vi "Monitor_Lithography_DAQ.vi"(8 "error in":errorcluster, 9 "Bmp Path":string, 10 "DAQ Channel":tag="Dev4/ai0:3", 11 "Application":refnum<k7>) -> (0 "error out":errorcluster)   [LabVIEW 2016]
panel:
  out "Tip Voltage":dbl
  out "Stop?":bool
  out "Position":cluster{dbl[], dbl[]}[](graph)=[{[8.144911482214924], [8.14400435631275]}, {[8.144911482214924, 8.144910315132138], [8.14400435631275, 8.144007987236977]}, {[8.144910315132138, 8.144959851312642], [8.144007987236977, 8.14406716265678]}, {[8.144959851312642, 8.144927562022207], [8.14406716265678, 8.144052941536904]}, {[8.144927562022207, 8.144947143077852], [8.144052941536904, 8.144056140208242]}, {[8.144947143077852, 8.144929852962496], [8.144056140208242, 8.144053935718532]}, {[8.144929852962496, 8.144989676761625], [8.144053935718532, 8.144058776950834]}, {[8.144989676761625, 8.144944549560549], [8.144058776950834, 8.144003621482849]}, {[8.144944549560549, 8.144922936916354], [8.144003621482849, 8.14404416680336]}, {[8.144922936916354, 8.144971954393386], [8.14404416680336, 8.144050045442585]}, {[8.144971954393386, 8.144984921979903], [8.144050045442585, 8.144040665555]}, {[8.144984921979903, 8.144920170497892], [8.144040665555, 8.144028389573094]}, {[8.144920170497892, 8.144943468928338], [8.144028389573094, 8.144053935718535]}, {[8.144943468928338, 8.144931754875186], [8.144053935718535, 8.144048835134507]}, {[8.144931754875186, 8.144938930273055], [8.144048835134507, 8.143980884981152]}, {[8.144938930273055, 8.144918657612802], [8.143980884981152, 8.144049353837962]}, {[8.144918657612802, 8.144969274425508], [8.144049353837962, 8.144027827644347]}, {[8.144969274425508, 8.144959721636772], [8.144027827644347, 8.144028648924827]}, {[8.144959721636772, 8.144974461460114], [8.144028648924827, 8.144024067044258]}, {[8.144974461460114, 8.144973596954344], [8.144024067044258, 8.144094956517216]}, {[8.144973596954344, 8.144982803940772], [8.144094956517216, 8.144038936543465]}, {[8.144982803940772, 8.14491061770916], [8.144038936543465, 8.14405030479431]}, {[8.14491061770916, 8.144952243661878], [8.14405030479431, 8.14406543364525]}, {[8.144952243661878, 8.144953886222842], [8.14406543364525, 8.144027395391467]}, {[8.144953886222842, 8.144932749056816], [8.144027395391467, 8.143989875841138]}, {[8.144932749056816, 8.144925616884233], [8.143989875841138, 8.144035478520392]}, {[8.144925616884233, 8.14495777649879], [8.144035478520392, 8.1440280005455]}, {[8.14495777649879, 8.144938195443158], [8.1440280005455, 8.143993593215939]}, {[8.144938195443158, 8.144955442333218], [8.143993593215939, 8.144091714620592]}, {[8.144955442333218, 8.144975931119921], [8.144091714620592, 8.14405363314152]}, {[8.144975931119921, 8.14493832511902], [8.14405363314152, 8.14401408200264]}, {[8.14493832511902, 8.14495574491024], [8.14401408200264, 8.14406050596237]}, {[8.14495574491024, 8.144944203758241], [8.14406050596237, 8.144046025490757]}, {[8.144944203758241, 8.144971522140503], [8.144046025490757, 8.14400941367149]}, {[8.144971522140503, 8.144928469753266], [8.14400941367149, 8.14405065059662]}, {[8.144928469753266, 8.144966118979456], [8.14405065059662, 8.14405553505421]}, {[8.144966118979456, 8.144937806415557], [8.14405553505421, 8.14403526239395]}, {[8.144937806415557, 8.144933310985564], [8.14403526239395, 8.144018101954456]}, {[8.144933310985564, 8.14493387291431], [8.144018101954456, 8.14404498808384]}, {[8.14493387291431, 8.144930933594702], [8.14404498808384, 8.144022510933878]}, {[8.144930933594702, 8.144931841325759], [8.144022510933878, 8.14399752671718]}, {[8.144931841325759, 8.144960499691958], [8.14399752671718, 8.144025493478775]}, {[8.144960499691958, 8.144941307663915], [8.144025493478775, 8.144049267387388]}, {[8.144941307663915, 8.144946408247947], [8.144049267387388, 8.1440012008667]}, {[8.144946408247947, 8.144917231178281], [8.1440012008667, 8.144034916591643]}, {[8.144917231178281, 8.144966378331182], [8.144034916591643, 8.14403746688366]}, {[8.144966378331182, 8.14490841321945], [8.14403746688366, 8.144000077009201]}, {[8.14490841321945, 8.144950514650342], [8.144000077009201, 8.144042913269997]}, {[8.144950514650342, 8.144938973498343], [8.144042913269997, 8.144022251582141]}, {[8.144938973498343, 8.144915026688574], [8.144022251582141, 8.143997094464304]}, {[8.144915026688574, 8.144913427352902], [8.143997094464304, 8.144011920738215]}, {[8.144913427352902, 8.144943468928338], [8.144011920738215, 8.144038936543463]}, {[8.144943468928338, 8.144950774002075], [8.144038936543463, 8.144024542522432]}, {[8.144950774002075, 8.144900027513504], [8.144024542522432, 8.144039973950383]}, {[8.144900027513504, 8.144928988456723], [8.144039973950383, 8.144039195895196]}, {[8.144928988456723, 8.144915415716165], [8.144039195895196, 8.14405194735527]}, {[8.144915415716165, 8.14489765012264], [8.14405194735527, 8.14400024991035]}, {[8.14489765012264, 8.144920343399047], [8.14400024991035, 8.144039325571056]}, {[8.144920343399047, 8.144949693369865], [8.144039325571056, 8.144044253253933]}, {[8.144949693369865, 8.144898860430716], [8.144044253253933, 8.144037337207797]}, {[8.144898860430716, 8.14497679562569], [8.144037337207797, 8.144061413693427]}, {[8.14497679562569, 8.144909580302238], [8.144061413693427, 8.144041659736635]}, {[8.144909580302238, 8.14492168338299], [8.144041659736635, 8.144023159313202]}, {[8.14492168338299, 8.144926783967016], [8.144023159313202, 8.144075807714463]}, {[8.144926783967016, 8.144996376681332], [8.144075807714463, 8.144012007188797]}, {[8.144996376681332, 8.144929507160185], [8.144012007188797, 8.14405004544258]}, {[8.144929507160185, 8.145012413263322], [8.14405004544258, 8.14407943863869]}, {[8.145012413263322, 8.144946970176695], [8.14407943863869, 8.144047970628739]}, {[8.144946970176695, 8.144920645976068], [8.144047970628739, 8.144028994727133]}, {[8.144920645976068, 8.144951768183708], [8.144028994727133, 8.144036256575587]}, {[8.144951768183708, 8.144971478915213], [8.144036256575587, 8.144038979768757]}, {[8.144971478915213, 8.144902750706668], [8.144038979768757, 8.144039844274518]}, {[8.144902750706668, 8.144973251152038], [8.144039844274518, 8.144061975622176]}, {[8.144973251152038, 8.14498885548115], [8.144061975622176, 8.144065649771688]}, {[8.14498885548115, 8.144957387471196], [8.144065649771688, 8.144028259897231]}, {[8.144957387471196, 8.144947705006599], [8.144028259897231, 8.14407745027542]}, {[8.144947705006599, 8.144953929448127], [8.14407745027542, 8.144061024665831]}, {[8.144953929448127, 8.144903269410129], [8.144061024665831, 8.144016761970521]}, {[8.144903269410129, 8.144941653466221], [8.144016761970521, 8.144070318102834]}, {[8.144941653466221, 8.144920256948469], [8.144070318102834, 8.144042178440095]}, {[8.144920256948469, 8.144934391617772], [8.144042178440095, 8.144027308940883]}, {[8.144934391617772, 8.144905517125128], [8.144027308940883, 8.14404338874817]}, {[8.144905517125128, 8.144976190471647], [8.14404338874817, 8.144069410371785]}, {[8.144976190471647, 8.144912562847137], [8.144069410371785, 8.143993204188344]}, {[8.144912562847137, 8.144963698363302], [8.143993204188344, 8.14406513106823]}, {[8.144963698363302, 8.144939276075362], [8.14406513106823, 8.144064828491208]}, {[8.144939276075362, 8.144948007583617], [8.144064828491208, 8.144054886674885]}, {[8.144948007583617, 8.14492427690029], [8.144054886674885, 8.14402268383503]}, {[8.14492427690029, 8.144954102349281], [8.14402268383503, 8.144067076206207]}, {[8.144954102349281, 8.144972775673866], [8.144067076206207, 8.144025839281083]}, {[8.144972775673866, 8.144915761518481], [8.144025839281083, 8.144049526739119]}, {[8.144915761518481, 8.144925833010676], [8.144049526739119, 8.144036991405484]}, {[8.144925833010676, 8.14495820875168], [8.144036991405484, 8.144011315584184]}, {[8.14495820875168, 8.144922893691064], [8.144011315584184, 8.144008203363418]}, {[8.144922893691064, 8.144907678389552], [8.144008203363418, 8.144014211678504]}, {[8.144907678389552, 8.144932619380949], [8.144014211678504, 8.14401641616821]}, {[8.144932619380949, 8.144914464759827], [8.14401641616821, 8.14404101135731]}, {[8.144914464759827, 8.144949347567556], [8.14404101135731, 8.144062796902652]}, {[8.144949347567556, 8.14494070250988], [8.144062796902652, 8.144028778600694]}, {[8.14494070250988, 8.144930069088938], [8.144028778600694, 8.144016070365904]}, {[8.144930069088938, 8.144888788938522], [8.144016070365904, 8.144020392894745]}, {[8.144888788938522, 8.144961926126483], [8.144020392894745, 8.144041832637786]}, {[8.144961926126483, 8.1449480940342], [8.144041832637786, 8.143984386229514]}, {[8.1449480940342, 8.144913297677041], [8.143984386229514, 8.144037121081352]}, {[8.144913297677041, 8.144947402429576], [8.144037121081352, 8.144033274030681]}, {[8.144947402429576, 8.144933094859123], [8.144033274030681, 8.144044426155087]}, {[8.144933094859123, 8.144935774827], [8.144044426155087, 8.144036040449144]}, {[8.144935774827, 8.144959289383886], [8.144036040449144, 8.14409002883434]}, {[8.144959289383886, 8.144931971001627], [8.14409002883434, 8.144005955648424]}, {[8.144931971001627, 8.144940270256994], [8.144005955648424, 8.144060116934776]}, {[8.144940270256994, 8.14496897184849], [8.144060116934776, 8.144052941536904]}, {[8.14496897184849, 8.144953756546977], [8.144052941536904, 8.144020263218877]}, {[8.144953756546977, 8.144940961861613], [8.144020263218877, 8.144020695471761]}, {[8.144940961861613, 8.144948915314673], [8.144020695471761, 8.144057955670357]}, {[8.144948915314673, 8.144953281068803], [8.144057955670357, 8.14403707785606]}, {[8.144953281068803, 8.144914335083962], [8.14403707785606, 8.144033533382416]}, {[8.144914335083962, 8.144987299370765], [8.144033533382416, 8.144030766963962]}, {[8.144987299370765, 8.144963828039167], [8.144030766963962, 8.144050520920752]}, {[8.144963828039167, 8.144963482236864], [8.144050520920752, 8.144027006363867]}, {[8.144963482236864, 8.144932273578641], [8.144027006363867, 8.144054497647284]}, {[8.144932273578641, 8.144970700860023], [8.144054497647284, 8.144073214197158]}, {[8.144970700860023, 8.144905819702148], [8.144073214197158, 8.144001806020734]}, {[8.144905819702148, 8.144957646822926], [8.144001806020734, 8.144050002217293]}, {[8.144957646822926, 8.144944981813431], [8.144050002217293, 8.14404740869999]}, {[8.144944981813431, 8.144936898684502], [8.14404740869999, 8.14403798558712]}, {[8.144936898684502, 8.144909407401085], [8.14403798558712, 8.144014384579659]}, {[8.144909407401085, 8.144961623549463], [8.144014384579659, 8.14405328733921]}, {[8.144961623549463, 8.144910488033295], [8.14405328733921, 8.144024326395991]}, {[8.144910488033295, 8.144942517971996], [8.144024326395991, 8.144046155166626]}, {[8.144942517971996, 8.14495820875168], [8.144046155166626, 8.144048489332201]}, {[8.14495820875168, 8.14493344066143], [8.144048489332201, 8.14401598391533]}, {[8.14493344066143, 8.144943814730647], [8.14401598391533, 8.14403932557106]}, {[8.144943814730647, 8.144969836354253], [8.14403932557106, 8.144098284864423]}, {[8.144969836354253, 8.144990584492684], [8.144098284864423, 8.14402605540752]}, {[8.144990584492684, 8.144929852962496], [8.14402605540752, 8.144051212525367]}, {[8.144929852962496, 8.145005367541316], [8.144051212525367, 8.144065692996977]}, {[8.145005367541316, 8.144951811408996], [8.144065692996977, 8.14404386422634]}, {[8.144951811408996, 8.1449167989254], [8.14404386422634, 8.14404287004471]}, {[8.1449167989254, 8.144952157211304], [8.14404287004471, 8.14408687338829]}, {[8.144952157211304, 8.144971997618672], [8.14408687338829, 8.14401836130619]}]
  # "For Local Variables"
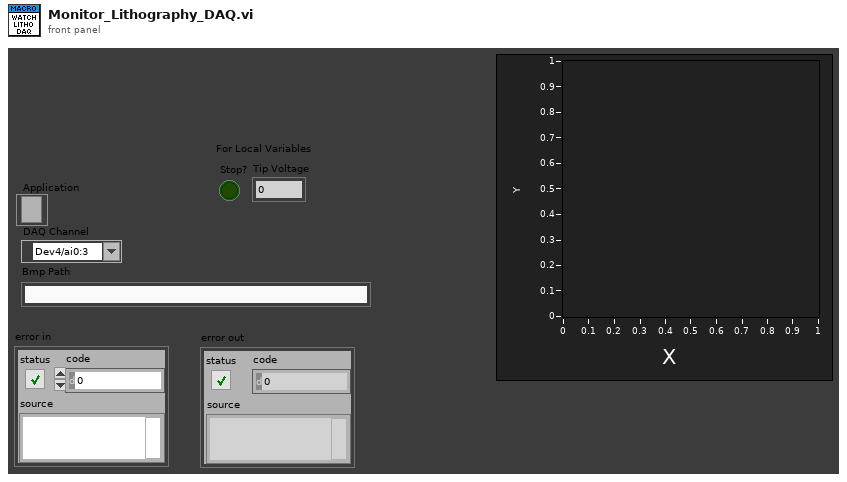
[diagram p1: front panel]
types:
  T1 = cluster{"Application":refnum<k7>, "Litho":refnum<k7>, "ZContr":refnum<k7>, "Scan":refnum<k7>}
  T2 = typedef "LVBoundsTypeDef.ctl" = cluster{"Width":u32, "Height":u32}
  T3 = typedef "LVPositionTypeDef.ctl" = cluster{"Left":i32, "Top":i32}
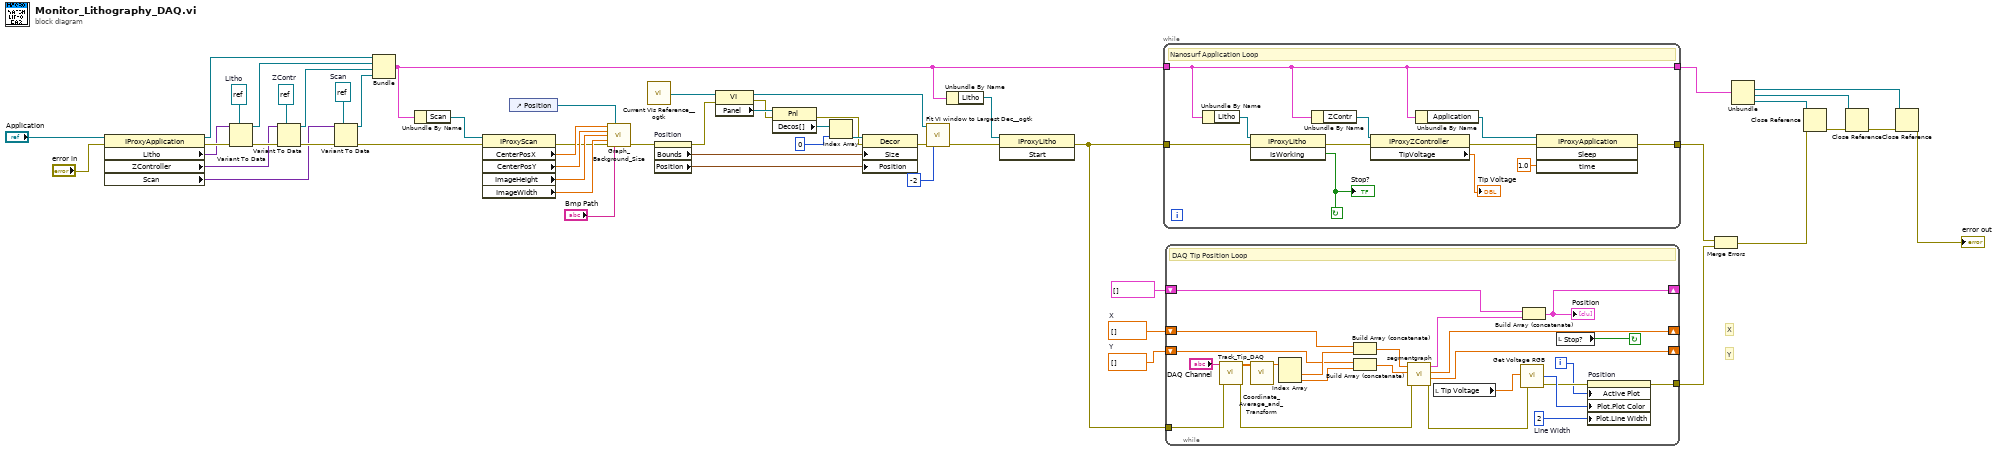
[diagram p0: block diagram]
diagram:
  w43 = dbl[] []  # Y
  w44 = dbl[] []  # X
  w46 = refnum<k7> refnum  # Scan
  w49 = refnum<k7> refnum  # ZContr
  w52 = refnum<k7> refnum  # Litho
  # "Y"
  # "X"
  n1 = property class="IProxyApplication"(reference="Application", error in="error in") -> (reference out=w36:refnum<k7>, error out=w54:errorcluster, "Litho"=w51:variant, "ZController"=w50:variant, "Scan"=w47:variant)
  n2 = Variant To Data(error in=w54, type=w52, Variant=w51) -> (data=w37:refnum<k7>, error out=w53:errorcluster)
  n3 = Variant To Data(error in=w53, type=w49, Variant=w50) -> (data=w35:refnum<k7>, error out=w48:errorcluster)
  n4 = Variant To Data(error in=w48, type=w46, Variant=w47) -> (data=w34:refnum<k7>, error out=w45:errorcluster)
  n5 = Bundle("Application"=w36, "Litho"=w37, "ZContr"=w35, "Scan"=w34) -> (w32:T1)  [unwired: 1 in]
  n6 = Unbundle By Name(w32) -> ("Scan"=w33:refnum<k7>)
  n7 = property class="IProxyScan"(reference=w33, error in=w45) -> (error out=w1:errorcluster, "CenterPosX"=w14:dbl, "CenterPosY"=w13:dbl, "ImageHeight"=w12:dbl, "ImageWidth"=w11:dbl)  [unwired: 1 out]
  n8 = control-ref of="Position"() -> (w15:refnum<vi>)
  n9 = call "Graph_Background_Size.vi"("CenterPosX"=w14, "XYGraph in"=w15, "CenterPosY"=w13, "Image Width"=w12, "Image Height"=w11, "error in (no error)"=w1, "Bmp Path"="Bmp Path") -> ("error out"=w17:errorcluster)  [unwired: 8 in]
  n10 = call <userlib>:"Current VIs Reference__ogtk.vi"() -> ("Current VI's reference"=w29:refnum<vi>)  [unwired: 5 in]
  n11 = property on="Position" class="XYGraph (strict)"(error in=w17) -> (error out=w20:errorcluster, "Bounds"=w24:T2, "Position"=w23:T3)  [unwired: 1 in, 1 out]
  n12 = property class="VI"(reference=w29, error in=w20) -> (reference out=w18:refnum<vi>, error out=w22:errorcluster, "Panel"=w28:refnum<vi>)
  n13 = property class="Pnl"(reference=w28, error in=w22) -> (error out=w21:errorcluster, "Decos[]"=w27:refnum<vi>[])  [unwired: 1 out]
  n14 = Index Array(array=w27, index=0) -> (element=w25:refnum<vi>)
  n15 = property class="Decor"(reference=w25, error in=w21, "Size"=w24, "Position"=w23) -> (error out=w19:errorcluster)  [unwired: 1 out]
  n16 = call <userlib>:"Fit VI window to Largest Dec__ogtk.vi"("error in (no error)"=w19, "border spacing (2 px)"=-2, "VI Ref (calling VI)"=w18) -> ("error out"=w16:errorcluster)  [unwired: 3 in, 1 out]
  n17 = Unbundle By Name(w32) -> ("Litho"=w31:refnum<k7>)
  n18 = invoke class="IProxyLitho" method="Start"(reference=w31, error in=w16) -> (error out=w41:errorcluster)  [unwired: 1 in, 2 out]
  n19 = while {
    tunnel: w41 -> [w66]
    tunnel: [w59] -> w39
    tunnel: w32 -> [w56]
    tunnel: [w56] -> w10
    stop <- w65 continue-if-true
    # "Nanosurf Application Loop"
    n20 = Unbundle By Name(w56) -> ("Litho"=w63:refnum<k7>)
    n21 = invoke class="IProxyLitho" method="IsWorking"(reference=w63, error in=w66) -> (error out=w64:errorcluster, "IsWorking"=w65:bool)  [unwired: 1 in, 1 out]
    "Stop?" <- w65
    n22 = Unbundle By Name(w56) -> ("ZContr"=w62:refnum<k7>)
    n23 = property class="IProxyZController"(reference=w62, error in=w64) -> (error out=w60:errorcluster, "TipVoltage"=→"Tip Voltage":dbl)  [unwired: 1 out]
    n24 = Unbundle By Name(w56) -> ("Application"=w58:refnum<k7>)
    n25 = invoke class="IProxyApplication" method="Sleep"(reference=w58, error in=w60, "time"=1.0) -> (error out=w59:errorcluster)  [unwired: 1 in, 3 out]
  }
  n26 = while {
    shift-right: [w76] -> _
    shift-left: w44 -> [w81]
    shift-right: [w75] -> _
    shift-left: w43 -> [w80]
    shift-right: [w88] -> _
    shift-left: cluster{dbl[], dbl[]}[] [] -> [w84]
    tunnel: w41 -> [w73]
    tunnel: [w70] -> w40
    i -> [w74]
    stop <- w69 continue-if-true
    w87 = u8 2  # Line Width
    # "DAQ Tip Position Loop"
    n27 = call "Track_Tip_DAQ.vi"("error in"=w73, "physical channels"="DAQ Channel") -> ("error out"=w72:errorcluster, "data"=w83:dbl[][])  [unwired: 8 in]
    n28 = call "Coordinate_Average_and_Transform.vi"("data"=w83) -> ("Array"=w82:dbl[])  [unwired: 10 in]
    n29 = Index Array(array=w82) -> (element #1=w90:dbl, element #2=w89:dbl)  [unwired: 2 in]
    n30 = Build Array (concatenate)(w81, w90) -> (w79:dbl[])
    n31 = Build Array (concatenate)(w80, w89) -> (w78:dbl[])
    n32 = call "segmentgraph.vi"("error in (no error)"=w72, "Y"=w78, "X"=w79) -> ("error out"=w71:errorcluster, "y out"=w75:dbl[], "xout"=w76:dbl[], "Segment"=w77:cluster{dbl[], dbl[]})  [unwired: 5 in]
    n33 = local read "Tip Voltage"() -> (w67:dbl)
    n34 = call <userlib>:"Get Voltage RGB.vi"("error in (no error)"=w71, "Voltage"=w67) -> ("error out"=w85:errorcluster, "RGB Value"=w86:u32)  [unwired: 1 in, 1 out]
    n35 = Build Array (concatenate)(w84, w77) -> (w88:cluster{dbl[], dbl[]}[])
    "Position" <- w88
    n36 = local read "Stop?"() -> (w69:bool)
    n37 = property on="Position" class="XYGraph (strict)"(error in=w85, "Active Plot"=w74, "Plot.Plot Color"=w86, "Plot.Line Width"=w87) -> (error out=w70:errorcluster)  [unwired: 1 in, 1 out]
  }
  n38 = Merge Errors(w39, w40) -> (w4:errorcluster)
  n39 = Unbundle(w10) -> ("Litho"=w7:refnum<k7>, "ZContr"=w8:refnum<k7>, "Scan"=w9:refnum<k7>)  [unwired: 1 out]
  n40 = Close Reference(reference=w9, error in (no error)=w4) -> (error out=w6:errorcluster)
  n41 = Close Reference(reference=w8, error in (no error)=w6) -> (error out=w5:errorcluster)
  n42 = Close Reference(reference=w7, error in (no error)=w5) -> (error out=→"error out":errorcluster)
